vi "4 Encoder PositionVelocity.vi"(0 "Encoder Inputs":T1={"Encoder In 0"="Chassis1/Mod4/DI0", "Encoder In 1"="Chassis1/Mod4/DI1", "Encoder In 2"="Chassis1/Mod4/DI2", "Encoder In 3"="Chassis1/Mod4/DI3"}, 2 "Encoder Interval (uSec)":u32=1000, 4 "Position Reset":bool) -> (7 "Encoder Packets":u64[](array[numeric]))   [LabVIEW 2010]
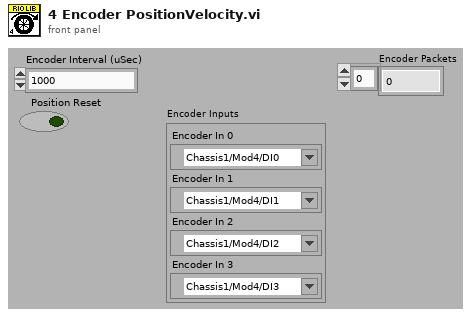
[diagram p1: front panel]
types:
  T1 = cluster{"Encoder In 0":refnum<k21>, "Encoder In 1":refnum<k21>, "Encoder In 2":refnum<k21>, "Encoder In 3":refnum<k21>}
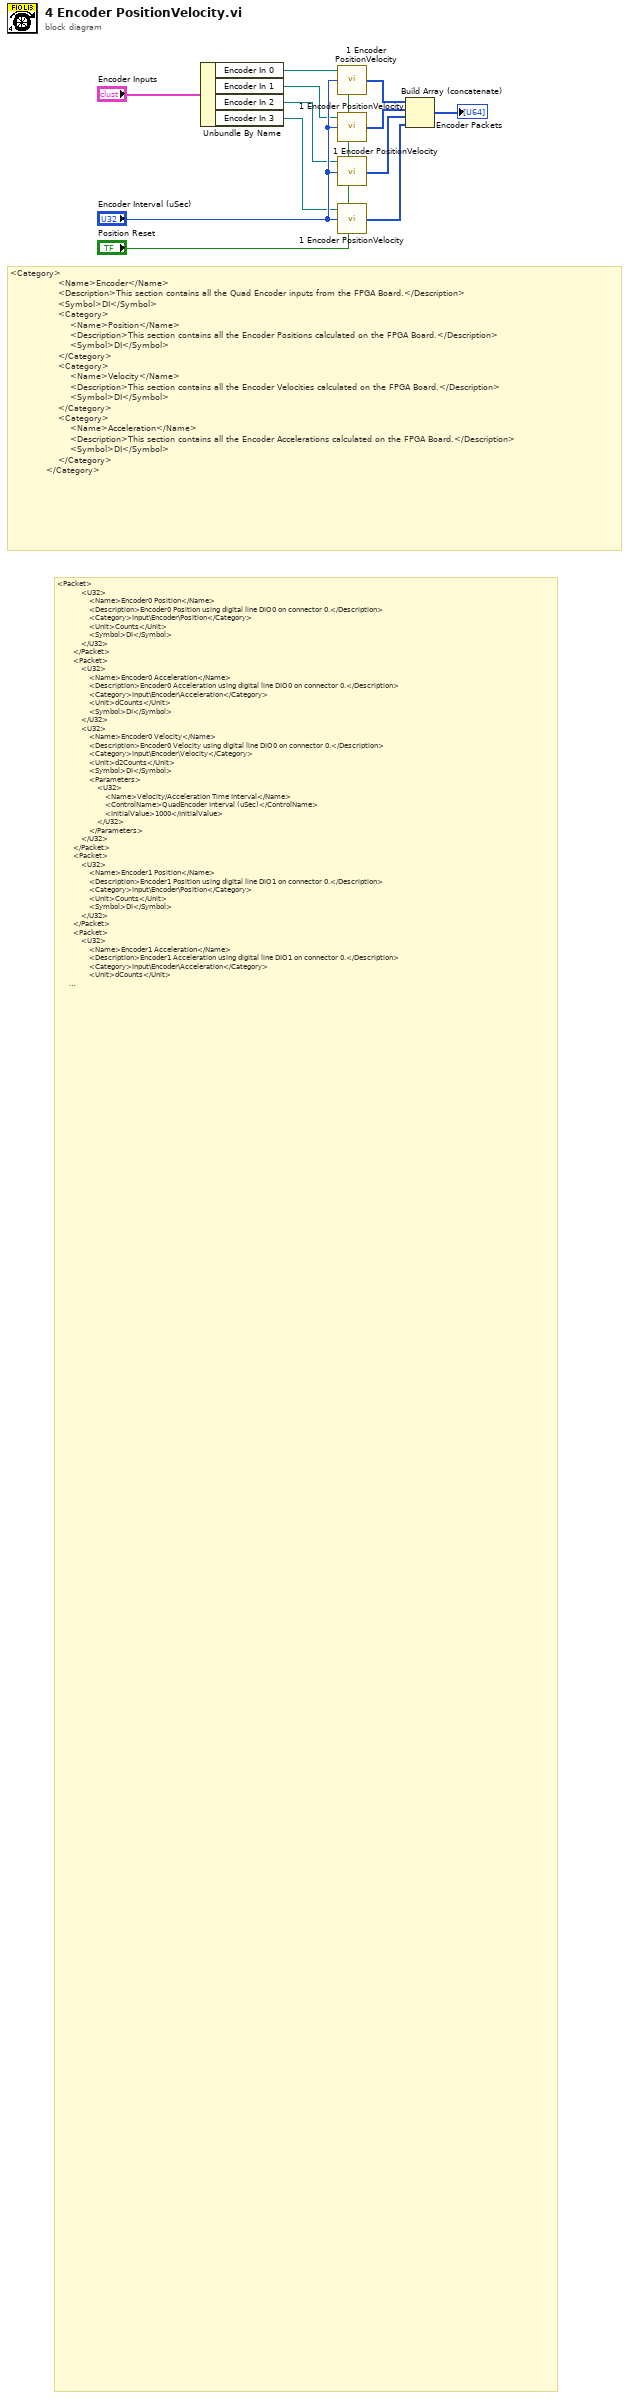
[diagram p0: block diagram]
diagram:
  # "<Category>\n                <Name>Encoder</Name>\n                <Description>This section contains all the Quad Encoder inputs from the FPGA Board.</Description>\n                <Symbol>DI</Symbol>\n                <Category>\n                    <Name>Position</Name>\n                    <Description>This section contains all the Encoder Positions calculated on the FPGA Board.</Description>\n                    <Symbol>DI</Symbol>\n                </Category>\n                <Category>\n                    <Name>Velocity</Name>\n                    <Description>This section contains all the Encoder Velocities calculated on the FPGA Board.</Description>\n                    <Symbol>DI</Symbol>\n                </Category>\n                <Category>\n                    <Name>Acceleration</Name>\n                    <Description>This section contains all the Encoder Accelerations calculated on the FPGA Board.</Description>\n                    <Symbol>DI</Symbol>\n                </Category>\n            </Category>"
  # "<Packet>\n            <U32>\n                <Name>Encoder0 Position</Name>\n                <Description>Encoder0 Position using digital line DIO0 on connector 0.</Description>\n                <Category>Input\\Encoder\\Position</Category>\n                <Unit>Counts</Unit>\n                <Symbol>DI</Symbol>\n            </U32>\n        </Packet>\n        <Packet>\n            <U32>\n                <Name>Encoder0 Acceleration</Name>\n                <Description>Encoder0 Acceleration using digital line DIO0 on connector 0.</Description>\n                <Category>Input\\Encoder\\Acceleration</Category>\n                <Unit>dCounts</Unit>\n                <Symbol>DI</Symbol>\n            </U32>\n            <U32>\n                <Name>Encoder0 Velocity</Name>\n                <Description>Encoder0 Velocity using digital line DIO0 on connector 0.</Description>\n                <Category>Input\\Encoder\\Velocity</Category>\n                <Unit>d2Counts</Unit>\n                <Symbol>DI</Symbol>\n                <Parameters>\n                    <U32>\n                        <Name>Velocity/Acceleration Time Interval</Name>\n                        <ControlName>QuadEncoder Interval (uSec)</ControlName>\n                        <InitialValue>1000</InitialValue>\n                    </U32>\n                </Parameters>\n            </U32>\n        </Packet>\n        <Packet>\n            <U32>\n                <Name>Encoder1 Position</Name>\n                <Description>Encoder1 Position using digital line DIO1 on connector 0.</Description>\n                <Category>Input\\Encoder\\Position</Category>\n                <Unit>Counts</Unit>\n                <Symbol>DI</Symbol>\n            </U32>\n        </Packet>\n        <Packet>\n            <U32>\n                <Name>Encoder1 Acceleration</Name>\n                <Description>Encoder1 Acceleration using digital line DIO1 on connector 0.</Description>\n                <Category>Input\\Encoder\\Acceleration</Category>\n                <Unit>dCounts</Unit>\n                <Symbol>DI</Symbol>\n            </U32>\n            <U32>\n                <Name>Encoder1 Velocity</Name>\n                <Description>Encoder1 Velocity using digital line DIO1 on connector 0.</Description>\n                <Category>Input\\Quad Encoder\\Velocity</Category>\n                <Unit>d2Counts</Unit>\n                <Symbol>DI</Symbol>\n                <Parameters>\n                    <U32>\n                        <Name>Velocity/Acceleration Time Interval</Name>\n                        <ControlName>QuadEncoder Interval (uSec)</ControlName>\n                        <InitialValue>1000</InitialValue>\n                    </U32>\n                </Parameters>\n            </U32>\n        </Packet>\n        <Packet>\n            <U32>\n                <Name>Encoder2 Position</Name>\n                <Description>Encoder2 Position using digital line DIO2 on connector 0.</Description>\n                <Category>Input\\Encoder\\Position</Category>\n                <Unit>Counts</Unit>\n                <Symbol>DI</Symbol>\n            </U32>\n        </Packet>\n        <Packet>\n            <U32>\n                <Name>Encoder2 Acceleration</Name>\n                <Description>Encoder2 Acceleration using digital line DIO2 on connector 0.</Description>\n                <Category>Input\\Encoder\\Acceleration</Category>\n                <Unit>dCounts</Unit>\n                <Symbol>DI</Symbol>\n            </U32>\n            <U32>\n                <Name>Encoder2 Velocity</Name>\n                <Description>Encoder2 Velocity using digital line DIO2 on connector 0.</Description>\n                <Category>Input\\Encoder\\Velocity</Category>\n                <Unit>d2Counts</Unit>\n                <Symbol>DI</Symbol>\n                <Parameters>\n                    <U32>\n                        <Name>Velocity/Acceleration Time Interval</Name>\n                        <ControlName>QuadEncoder Interval (uSec)</ControlName>\n                        <InitialValue>1000</InitialValue>\n                    </U32>\n                </Parameters>\n            </U32>\n        </Packet>\n        <Packet>\n            <U32>\n                <Name>Encoder3 Position</Name>\n                <Description>Encoder3 Position using digital line DIO3 on connector 0.</Description>\n                <Category>Input\\Encoder\\Position</Category>\n                <Unit>Counts</Unit>\n                <Symbol>DI</Symbol>\n            </U32>\n        </Packet>\n        <Packet>\n            <U32>\n                <Name>Encoder3 Acceleration</Name>\n                <Description>Encoder3 Acceleration using digital line DIO3 on connector 0.</Description>\n                <Category>Input\\Encoder\\Acceleration</Category>\n                <Unit>dCounts</Unit>\n                <Symbol>DI</Symbol>\n            </U32>\n            <U32>\n                <Name>Encoder3 Velocity</Name>\n                <Description>Encoder3 Velocity using digital line DIO3 on connector 0.</Description>\n                <Category>Input\\Quad Encoder\\Velocity</Category>\n                <Unit>d2Counts</Unit>\n                <Symbol>DI</Symbol>\n                <Parameters>\n                    <U32>\n                        <Name>Velocity/Acceleration Time Interval</Name>\n                        <ControlName>QuadEncoder Interval (uSec)</ControlName>\n                        <InitialValue>1000</InitialValue>\n                    </U32>\n                </Parameters>\n            </U32>\n        </Packet>"
  n1 = Unbundle By Name("Encoder Inputs") -> ("Encoder In 0"=w4:refnum<k21>, "Encoder In 1"=w3:refnum<k21>, "Encoder In 2"=w2:refnum<k21>, "Encoder In 3"=w1:refnum<k21>)
  n2 = call <userlib>:"1 Encoder PositionVelocity.vi"("Encoder Input"=w4, "Encoder Interval (uSec)"="Encoder Interval (uSec)", "Position Reset"="Position Reset") -> ("Encoder Packets"=w11:u64[])  [unwired: 6 in]
  n3 = call <userlib>:"1 Encoder PositionVelocity.vi"("Encoder Input"=w3, "Encoder Interval (uSec)"="Encoder Interval (uSec)", "Position Reset"="Position Reset") -> ("Encoder Packets"=w12:u64[])  [unwired: 6 in]
  n4 = call <userlib>:"1 Encoder PositionVelocity.vi"("Encoder Input"=w2, "Encoder Interval (uSec)"="Encoder Interval (uSec)", "Position Reset"="Position Reset") -> ("Encoder Packets"=w5:u64[])  [unwired: 6 in]
  n5 = call <userlib>:"1 Encoder PositionVelocity.vi"("Encoder Input"=w1, "Encoder Interval (uSec)"="Encoder Interval (uSec)", "Position Reset"="Position Reset") -> ("Encoder Packets"=w6:u64[])  [unwired: 6 in]
  n6 = Build Array (concatenate)(w11, w12, w5, w6) -> (→"Encoder Packets":u64[])
